vi "Add Item to Tree.vi"(6 "Display Text Override":string, 7 "Child only? (F)":bool, 8 "error in (no error)":errorcluster, 9 "Parent Tag":string, 10 "Data Item":refnum<class "Data Item.lvclass">, 11 "Tree Manager in":refnum<class "Tree Manager.lvclass">) -> (0 "error out":errorcluster, 2 "New Tag":string, 3 "Tree Manager out":refnum<class "Tree Manager.lvclass">)   [LabVIEW 2023, in "VILab.lvlib" / "Tree Manager.lvclass"]
uses:
  Tree Manager.lvclass
  Data Item/Data Item.lvclass
  Tree Manager.lvclass/Tree Manager.ctl
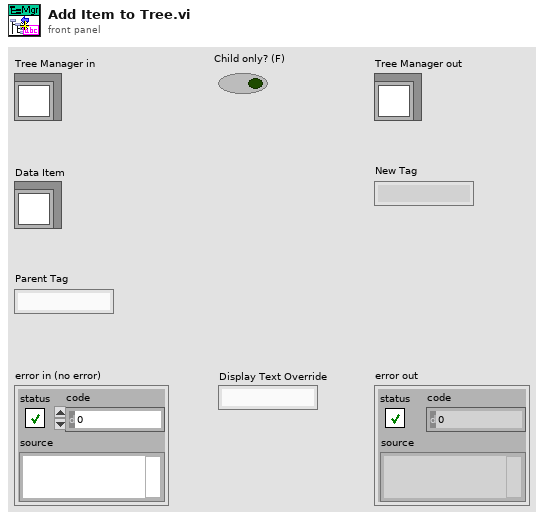
[diagram p1: front panel]
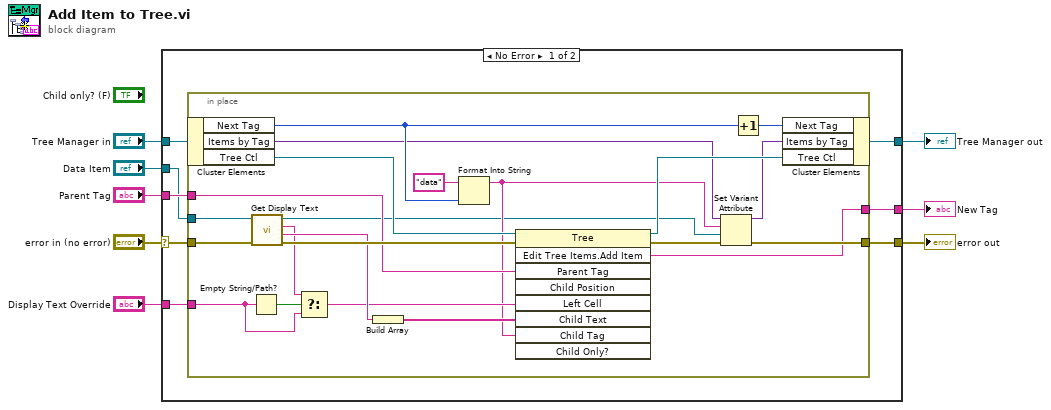
[diagram p0: block diagram]
diagram:
  n1 = case shown="No Error" "error in (no error)" {
    selector: "error in (no error)" -> [w16 w40]
    tunnel: [w15 w40] -> w7
    tunnel: [w11 w39] -> w5
    tunnel: "Tree Manager in" -> [w14 w39]
    tunnel: "Data Item" -> [w9 _]
    tunnel: "Parent Tag" -> [w13 _]
    tunnel: [w12 _] -> w2
    tunnel: "Display Text Override" -> [w10 _]
    frame No Error {
      n2 = in-place {
        in-place-border: w9 -> [w34]
        in-place-border: w16 -> [w38]
        in-place-border: w13 -> [w32]
        in-place-border: [w24] -> w12
        in-place-border: w10 -> [w18]
        in-place-border: [w35] -> w15
        n3 = in-place-cluster #1(w14) -> ("Next Tag"=w26:u64, "Items by Tag"=w21:variant, "Tree Ctl"=w33:refnum<vi>)
        n4 = Empty String/Path?(string/path=w18) -> (empty?=w17:bool)
        n5 = call-dynamic "Get Display Text.vi"("error in (no error)"=w38, "Data Item in"=w34) -> ("error out"=w36:errorcluster, "Detail Text"=w31:string, "Display Name"=w20:string, "Data Item out"=w19:refnum<class "Data Item.lvclass">)  [unwired: 6 in]
        n6 = Select(t=w20, s=w17, f=w18) -> (s? t:f=w23:string)
        n7 = Build Array(w31) -> (w30:string[])
        n8 = Format Into String(initial string="data", w26) -> (resulting string=w22:string)  [unwired: 2 in, 1 out]
        n9 = invoke class="Tree" method="Edit Tree Items.Add Item"(reference=w33, error in=w36, "Parent Tag"=w32, "Left Cell"=w23, "Child Text"=w30, "Child Tag"=w22) -> (reference out=w29:refnum<vi>, error out=w37:errorcluster, "Edit Tree Items:Add Item"=w24:string)  [unwired: 3 in, 6 out]
        n10 = Set Variant Attribute(Variant=w21, name=w22, value=w19, error in=w37) -> (Variant out=w28:variant, error out=w35:errorcluster)  [unwired: 1 out]
        n11 = Increment(x=w26) -> (x+1=w27:u64)
        n12 = in-place-cluster #1("Next Tag"=w27, "Items by Tag"=w28, "Tree Ctl"=w29) -> (w11:refnum<class "Tree Manager.lvclass">)
      }
    }
    frame Error {
    }
  }
  "error out" <- w7
  "Tree Manager out" <- w5
  "New Tag" <- w2
